vi "daqio_Replace_File.vi"(8 "error in":errorcluster, 9 "File to be uploaded":path, 10 "asset ID to replace":string, 11 "daq.io type in":T1={"daq.io ref"=refnum, "daq.io API Base"="http://dashboard.daq.io/api/v1", "Device Key"="", "Account ID"="", "online"=TRUE, "SSL"=TRUE, "buffer"=TRUE}) -> (0 "error out":errorcluster, 3 "daq.io type out":T1={"daq.io ref"=refnum, "daq.io API Base"="http://dashboard.daq.io/api/v1", "Device Key"="", "Account ID"="", "online"=TRUE, "SSL"=TRUE, "buffer"=TRUE})   [LabVIEW 2013, in "daqio minimal.lvlib"]
doc: "This VI uploads a new user file. It can be any file type. However, images and CSV files will be treated specially on daq.io, therefore make sure to select the correct file type, if you want features like the image preview to work. For PDF files, please select binary. \nThe VI will return the unique file ID that can be used to retrieve the file later and link it to a device."
uses:
  daqio minimal.lvlib
  _typedefs/daqio-Type.ctl
  <vilib>/httpClient/ClientHandle.ctl
  <vilib>/httpClient/MultipartData.ctl
  _typedefs/daqio-Credentials-FGV.ctl
  <vilib>/Easy HTTP Client/Easy HTTP.lvlib
  <vilib>/httpClient/LabVIEWHTTPClient.lvlib
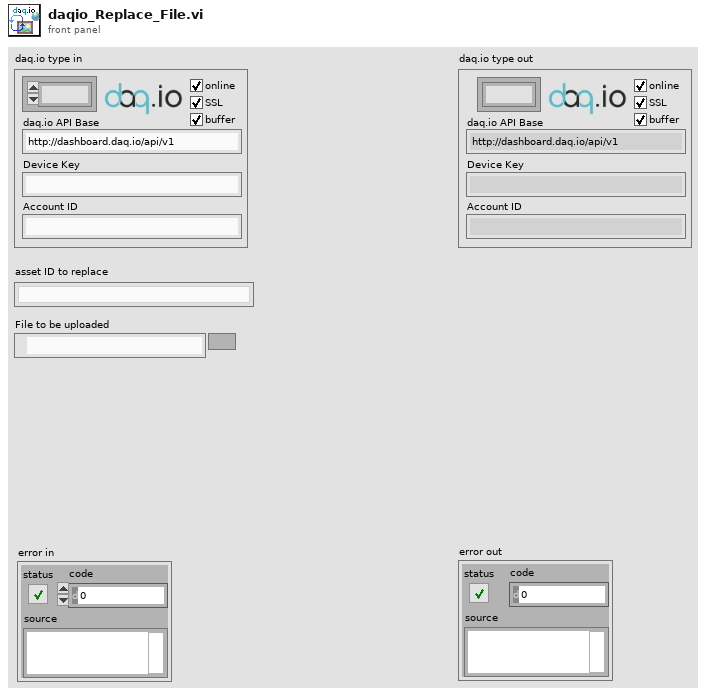
[diagram p1: front panel]
types:
  T1 = typedef "daqio minimal.lvlib/daqio-Type.ctl" = cluster{"daq.io ref":T2, "daq.io API Base":string, "Device Key":string, "Account ID":string, "online":bool, "SSL":bool, "buffer":bool}
  T2 = typedef "LabVIEWHTTPClient.lvlib/ClientHandle.ctl" = refnum<k1>
  T3 = typedef "daqio minimal.lvlib/daqio-Credentials-FGV.ctl" = enum16{"Generate", "Read"}
  T4 = typedef "LabVIEWHTTPClient.lvlib/MultipartData.ctl" = cluster{"Name":string, "Value":string, "File":path, "Filename":string, "MIME type":string}
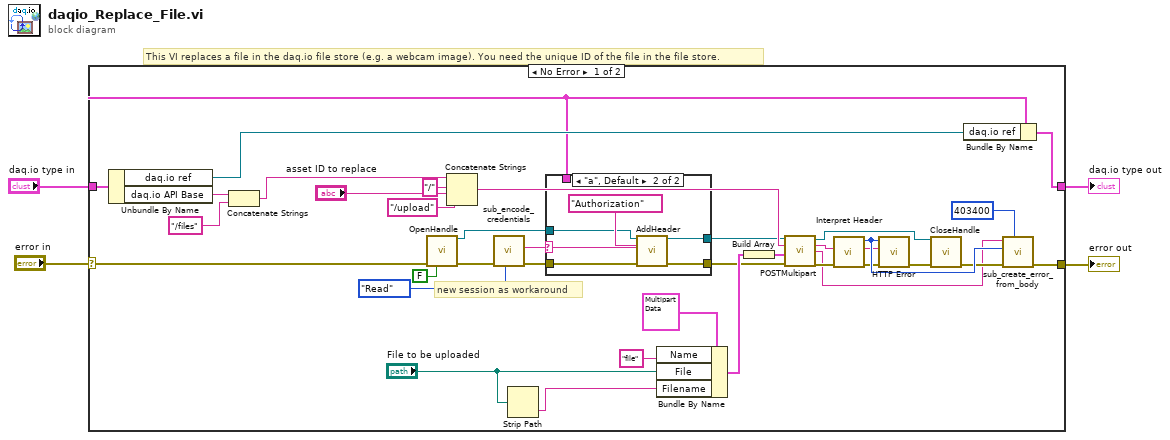
[diagram p0: block diagram]
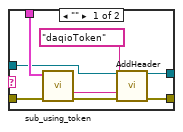
[diagram p2: hidden frame]
diagram:
  # "This VI replaces a file in the daq.io file store (e.g. a webcam image). You need the unique ID of the file in the file store."
  n1 = case shown="No Error" "error in" {
    selector: "error in" -> [w15 w55]
    tunnel: "daq.io type in" -> [w9 w56]
    tunnel: [w37 w56] -> w3
    tunnel: [w39 w55] -> w2
    frame No Error {
      # "new session as workaround"
      n2 = Unbundle By Name(w9) -> ("daq.io ref"=w13:T2, "daq.io API Base"=w38:string)
      n3 = Concatenate Strings(w38, "/files") -> (w36:string)
      n4 = call <vilib>:"OpenHandle.vi"("error in (no error)"=w15, "verify server(true)"=FALSE) -> ("client handle out"=w7:T2, "error out"=w22:errorcluster)  [unwired: 12 in]
      n5 = Concatenate Strings(w36, "/" ("string"), "asset ID to replace", "/upload" ("string")) -> (w31:string)
      n6 = call "sub_encode_credentials.vi"("Command"=daqio-Credentials-FGV."Read", "error in"=w22) -> ("error out"=w10:errorcluster, "Stored Credentials"=w11:string)  [unwired: 7 in, 1 out]
      n7 = Strip Path(path="File to be uploaded") -> (name=w14:string)  [unwired: 1 out]
      n8 = case shown="\"a\", Default" w11 {
        selector: w11 -> [_ w51]
        tunnel: [w45 w53] -> w5
        tunnel: [w44 w52] -> w8
        tunnel: w10 -> [w43 w50]
        tunnel: w9 -> [w42 _]
        tunnel: w7 -> [w41 w49]
        frame "" {
          n9 = call "sub_using_token.vi"("error in (no error)"=w43, "daq.io type in"=w42) -> ("error out"=w46:errorcluster, "Token ID"=w47:string)  [unwired: 6 in, 2 out]
          n10 = call <vilib>:"AddHeader.vi"("client handle"=w41, "header"="daqioToken", "value"=w47, "error in (no error)"=w46) -> ("client handle out"=w45:T2, "error out"=w44:errorcluster)  [unwired: 10 in]
        }
        frame "a", Default {
          n11 = call <vilib>:"AddHeader.vi"("client handle"=w49, "header"="Authorization", "value"=w51, "error in (no error)"=w50) -> ("client handle out"=w53:T2, "error out"=w52:errorcluster)  [unwired: 10 in]
        }
      }
      n12 = Bundle By Name(cluster=T4 {"Name"="", "Value"="", "File"=path "", "Filename"="", "MIME type"="application/octet-stream"} ("Element"), "Name"="file", "File"="File to be uploaded", "Filename"=w14) -> (w26:T4)
      n13 = Build Array(w26) -> (w25:T4[])
      n14 = call <vilib>:"POSTMultipart.vi"("client handle"=w5, "url"=w31, "data"=w25, "error in (no error)"=w8) -> ("client handle out"=w20:T2, "headers"=w28:string, "body"=w17:string, "error out"=w27:errorcluster)  [unwired: 8 in]
      n15 = call <vilib>:"Interpret Header.vi"("error in (no error)"=w27, "Header"=w28) -> ("error out"=w29:errorcluster, "HTTP Response"=w30:string, "HTTP Code"=w32:i32)  [unwired: 5 in, 2 out]
      n16 = call <vilib>:"HTTP Error.vi"("error in (no error)"=w29, "HTTP Response"=w30, "HTTP Code"=w32) -> ("error out"=w21:errorcluster)  [unwired: 8 in]
      n17 = call <vilib>:"CloseHandle.vi"("client handle"=w20, "error in (no error)"=w21) -> ("error out"=w19:errorcluster)  [unwired: 13 in]
      n18 = Bundle By Name(cluster=w9, "daq.io ref"=w13) -> (w37:T1)
      n19 = call "sub_create_error_from_body.vi"("error code"=403400, "error in (no error)"=w19, "http code"=w32, "body"=w17) -> ("error out"=w39:errorcluster)  [unwired: 7 in]
    }
    frame Error {
    }
  }
  "error out" <- w2
  "daq.io type out" <- w3
